vi "Handle Command.vi"(8 "error in (no error)":errorcluster, 9 "params in":variant, 10 "command":string, 11 "Instrument in":refnum<class "Instrument.lvclass">) -> (0 "error out":errorcluster, 1 "processed data":variant, 2 "command out":string, 3 "Instrument out":refnum<class "Instrument.lvclass">)   [LabVIEW 2019, in "Instrument.lvlib" / "Instrument.lvclass"]
doc: "Override to add additional commands supported by your Instrument."
uses:
  Instrument.lvclass
  Typedefs/Instrument.Commands--Enum.ctl
  Typedefs/Instrument.ProtectedCommands--Enum.ctl
  Typedefs/Instrument.SET--cluster.ctl
  Typedefs/Instrument.GET--cluster.ctl
  acbd13c6-77b8-4678-afb4-11360eefb496.vi
  94f5b594-5f3e-4275-9402-05a479f08510.vi
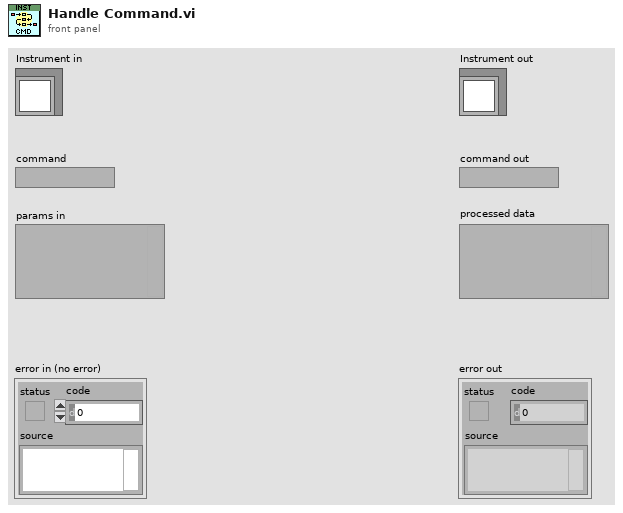
[diagram p1: front panel]
types:
  T1 = typedef "Instrument.lvlib/Instrument.lvclass/Instrument.ProtectedCommands--Enum.ctl" = enum16{"setConfiguration", "setIDN", "setAll", "setAllData"}
  T2 = typedef "Instrument.lvlib/Instrument.lvclass/Instrument.Commands--Enum.ctl" = enum16{"ACK", "HELP", "IDN", "getAll", "getAllData"}
  T3 = typedef "Instrument.lvlib/Instrument.lvclass/Instrument.GET--cluster.ctl" = cluster{"parameter":string, "Data":variant}
  T4 = typedef "Instrument.lvlib/Instrument.lvclass/Instrument.SET--cluster.ctl" = cluster{"parameter":string, "Data":variant}
  T5 = typedef "Instrument.lvlib/Instrument.lvclass/Instrument.IDN--cluster.ctl" = cluster{"vendor":string, "model":string, "serial":string, "firmware":string}
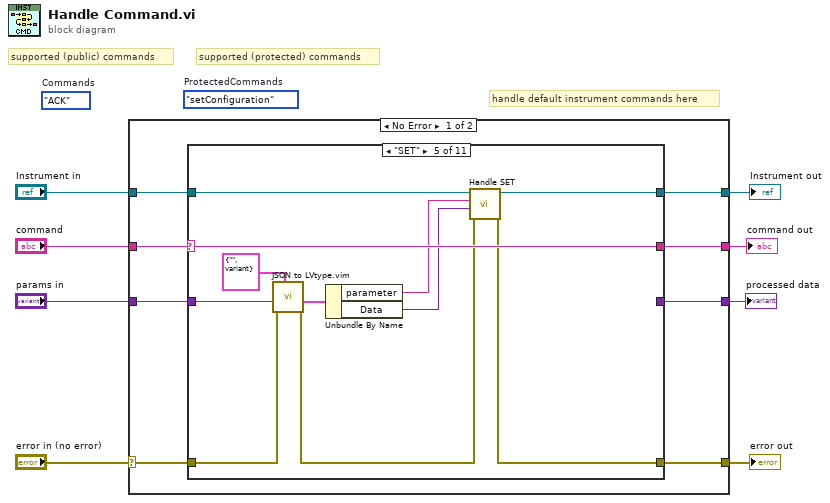
[diagram p0: block diagram]
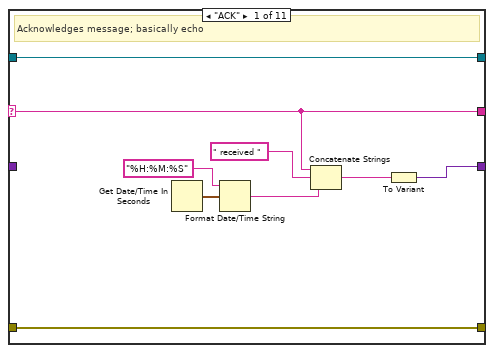
[diagram p2: hidden frame]
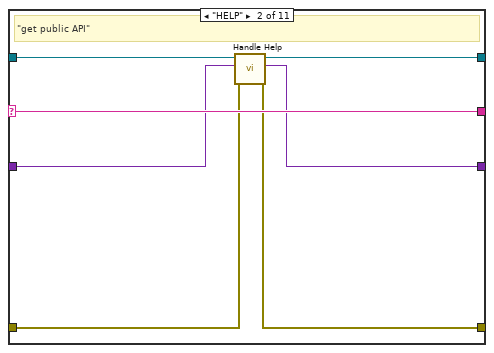
[diagram p3: hidden frame]
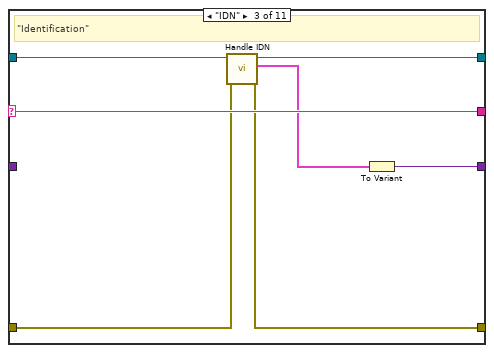
[diagram p4: hidden frame]
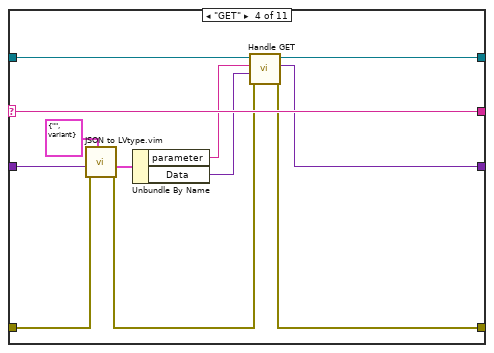
[diagram p5: hidden frame]
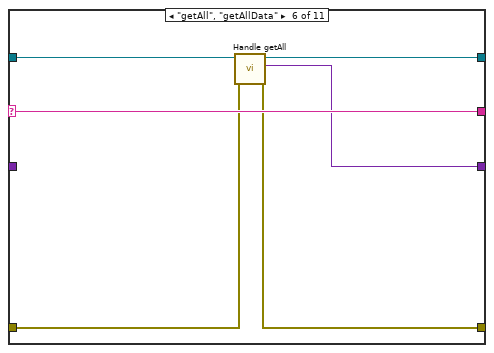
[diagram p6: hidden frame]
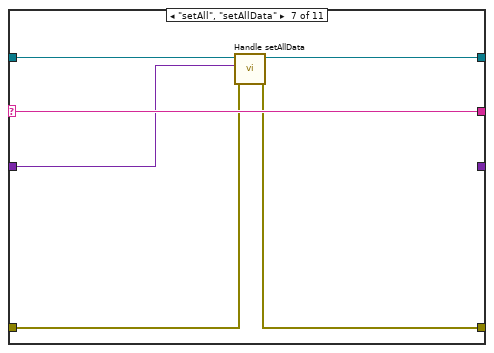
[diagram p7: hidden frame]
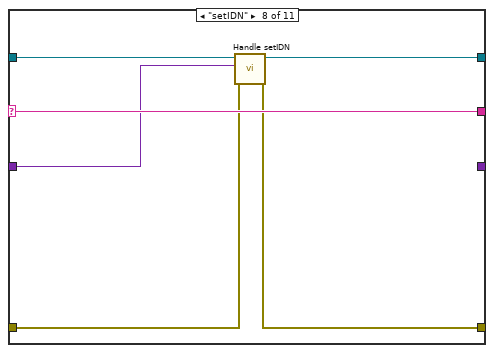
[diagram p8: hidden frame]
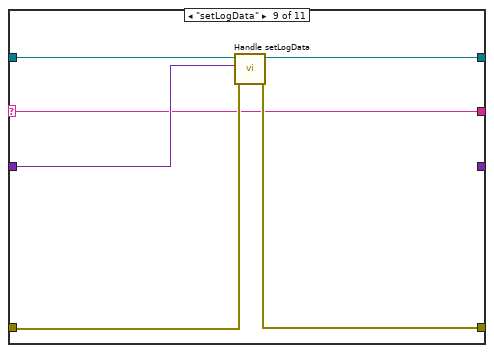
[diagram p9: hidden frame]
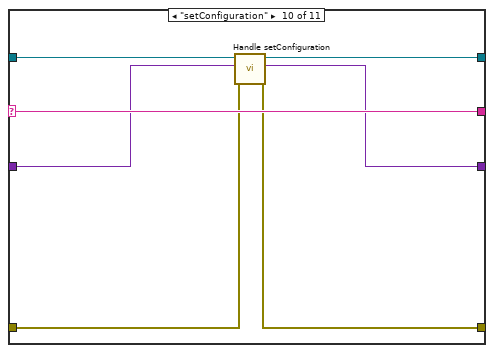
[diagram p10: hidden frame]
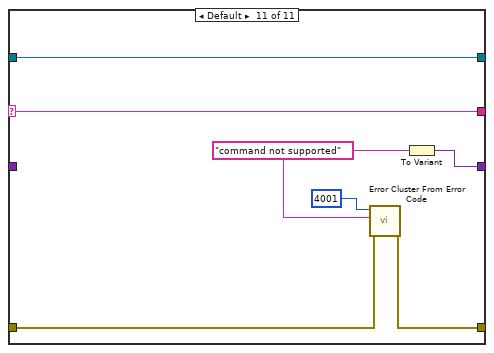
[diagram p11: hidden frame]
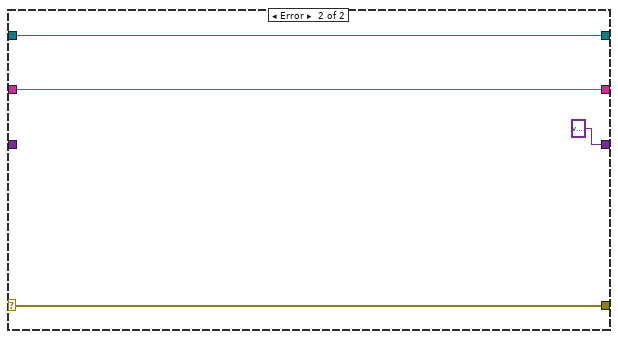
[diagram p12: hidden frame]
diagram:
  (unwired) Instrument.ProtectedCommands--Enum."setConfiguration"  # ProtectedCommands
  (unwired) Instrument.Commands--Enum."ACK"  # Commands
  # "supported (protected) commands"
  # "supported (public) commands"
  # "handle default instrument commands here"
  n1 = case shown="No Error" "error in (no error)" {
    selector: "error in (no error)" -> [w13 w103]
    tunnel: [w12 w103] -> w7
    tunnel: [w15 w102] -> w5
    tunnel: "Instrument in" -> [w16 w102]
    tunnel: "command" -> [w10 w101]
    tunnel: [w14 variant ("error message (\"\")")] -> w4
    tunnel: "params in" -> [w9 _]
    tunnel: [w11 w101] -> w1
    frame No Error {
      n2 = case shown="\"SET\"" w10 {
        selector: w10 -> [w19 w30 w39 w51 w62 w68 w74 w80 w81 w92 w97]
        tunnel: w16 -> [w25 w32 w36 w49 w60 w65 w73 w78 w86 w89 w99]
        tunnel: [w25 w31 w37 w50 w61 w64 w72 w76 w85 w88 w99] -> w15
        tunnel: [w17 w27 w38 w47 _ w63 _ _ _ w87 w98] -> w14
        tunnel: w13 -> [w22 w29 w33 w45 w56 w67 w71 w79 w83 w91 w95]
        tunnel: [w22 w28 w34 w48 w59 w66 w70 w77 w82 w90 w94] -> w12
        tunnel: [w19 w30 w39 w51 w62 w68 w74 w80 w81 w92 w97] -> w11
        tunnel: w9 -> [_ w26 _ w42 w55 _ w69 w75 w84 w87 _]
        frame "ACK" {
          # "Acknowledges message; basically echo"
          n3 = Get Date/Time In Seconds() -> (seconds since 1Jan1904=w23:timestamp)
          n4 = Format Date/Time String(time format string (%c)="%H:%M:%S", seconds (now)=w23) -> (date/time string=w24:string)  [unwired: 1 in]
          n5 = Concatenate Strings(w19, " received " ("data"), w24) -> (w21:string)
          n6 = To Variant(anything=w21) -> (Variant=w17:variant)
        }
        frame "HELP" {
          # "\"get public API\""
          n7 = call "Handle Help.vi"("error in (no error)"=w29, "Command"=w26, "Instrument in"=w32) -> ("error out"=w28:errorcluster, "Help"=w27:variant, "Instrument out"=w31:refnum<class "Instrument.lvclass">)  [unwired: 6 in]
        }
        frame "IDN" {
          # "\"Identification\""
          n8 = call "Handle IDN.vi"("error in (no error)"=w33, "Instrument in"=w36) -> ("error out"=w34:errorcluster, "IDN"=w35:T5, "Instrument out"=w37:refnum<class "Instrument.lvclass">)  [unwired: 7 in]
          n9 = To Variant(anything=w35) -> (Variant=w38:variant)
        }
        frame "GET" {
          n10 = call "JSON to LVtype.vim"("type"=T3 {"parameter"="", "Data"=variant} ("GET"), "error in (no error)"=w45, "JSON Data in"=w42) -> ("error out"=w46:errorcluster, "Data out"=w40:T3)  [unwired: 7 in]
          n11 = Unbundle By Name(w40) -> ("parameter"=w44:string, "Data"=w43:variant)
          n12 = call-dynamic "Handle GET.vi"("error in (no error)"=w46, "data"=w43, "parameter"=w44, "Instrument in"=w49) -> ("error out"=w48:errorcluster, "data out"=w47:variant, "Instrument out"=w50:refnum<class "Instrument.lvclass">)  [unwired: 5 in]
        }
        frame "SET" {
          n13 = call "JSON to LVtype.vim"("type"=T4 {"parameter"="", "Data"=variant} ("GETSET"), "error in (no error)"=w56, "JSON Data in"=w55) -> ("error out"=w54:errorcluster, "Data out"=w53:T4)  [unwired: 7 in]
          n14 = Unbundle By Name(w53) -> ("parameter"=w58:string, "Data"=w57:variant)
          n15 = call-dynamic "Handle SET.vi"("error in (no error)"=w54, "data"=w57, "parameter"=w58, "Instrument in"=w60) -> ("error out"=w59:errorcluster, "Instrument out"=w61:refnum<class "Instrument.lvclass">)  [unwired: 5 in, 1 out]
        }
        frame "getAll", "getAllData" {
          n16 = call-dynamic "Handle getAll.vi"("error in (no error)"=w67, "Instrument in"=w65) -> ("error out"=w66:errorcluster, "getAll"=w63:variant, "Instrument out"=w64:refnum<class "Instrument.lvclass">)  [unwired: 7 in]
        }
        frame "setAll", "setAllData" {
          n17 = call-dynamic "Handle setAllData.vi"("error in (no error)"=w71, "AllData"=w69, "Instrument in"=w73) -> ("error out"=w70:errorcluster, "Instrument out"=w72:refnum<class "Instrument.lvclass">)  [unwired: 7 in]
        }
        frame "setIDN" {
          n18 = call "Handle setIDN.vi"("error in (no error)"=w79, "IDN"=w75, "Instrument in"=w78) -> ("error out"=w77:errorcluster, "Instrument out"=w76:refnum<class "Instrument.lvclass">)  [unwired: 7 in]
        }
        frame "setLogData" {
          n19 = call "Handle setLogData.vi"("error in (no error)"=w83, "LogData"=w84, "Instrument in"=w86) -> ("error out"=w82:errorcluster, "Instrument out"=w85:refnum<class "Instrument.lvclass">)  [unwired: 7 in]
        }
        frame "setConfiguration" {
          n20 = call-dynamic "Handle setConfiguration.vi"("error in (no error)"=w91, "setConfiguration"=w87, "Instrument in"=w89) -> ("error out"=w90:errorcluster, "Instrument out"=w88:refnum<class "Instrument.lvclass">)  [unwired: 7 in]
        }
        frame Default {
          w93 = "command not supported" ("error message (\"\")")
          n21 = call <vilib>:"Error Cluster From Error Code.vi"("error in (no error)"=w95, "error message (\"\")"=w93, "error code (0)"=4001) -> ("error out"=w94:errorcluster)  [unwired: 6 in]
          n22 = To Variant(anything=w93) -> (Variant=w98:variant)
        }
      }
    }
    frame Error {
    }
  }
  "error out" <- w7
  "Instrument out" <- w5
  "processed data" <- w4
  "command out" <- w1
